vi "Delacor_lib_QMH_Error Handler - Framework Loop.vi"(6 "Error Message Name (\"Error\")":string="Error", 8 "error in":errorcluster, 10 "Ignore Errors (Runtime)":i32[](array[numeric]), 11 "Message Queue in":refnum<class "RQMHMessageQueue.lvclass">) -> (0 "dup error in":errorcluster, 3 "Message Queue out":refnum<class "RQMHMessageQueue.lvclass">)   [LabVIEW 2024, in "RQMHMessageQueue.lvclass"]
doc: "Process an error that occurred in the Event Handling Loop, either by ignoring it, or generating an \"Error\" message.\n____\nDQMH Framework: Palette 7.1.0.1503\nCopyright (c) 2025, DQMH Consortium"
uses:
  RQMHMessageQueue.lvclass
  RQMHMessageQueue.lvclass/RQMHMessageQueue.ctl
  Delacor_lib_QMH_Set Error Debug.vi
  Delacor_lib_QMH_Get Error Debug.vi
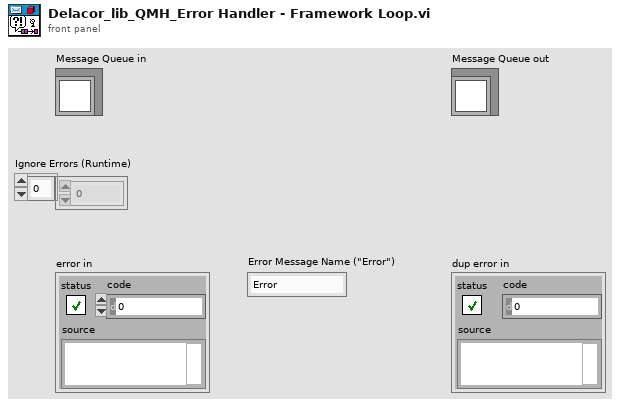
[diagram p1: front panel]
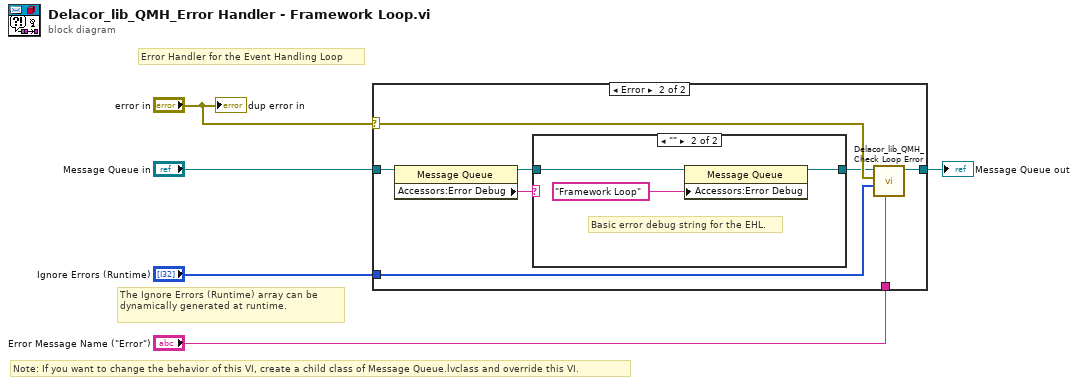
[diagram p0: block diagram]
diagram:
  # "Note: If you want to change the behavior of this VI, create a child class of Message Queue.lvclass and override this VI."
  # "The Ignore Errors (Runtime) array can be dynamically generated at runtime."
  # "Error Handler for the Event Handling Loop"
  n1 = case shown="Error" "error in" {
    selector: "error in" -> [_ w14]
    tunnel: "Message Queue in" -> [w6 w13]
    tunnel: "Ignore Errors (Runtime)" -> [_ w12]
    tunnel: [w6 w11] -> w2
    tunnel: "Error Message Name (\"Error\")" -> [_ w10]
    frame No Error {
    }
    frame Error {
      n2 = property class="Message Queue"(reference=w13) -> (reference out=w8:refnum<class "RQMHMessageQueue.lvclass">, "Accessors:Error Debug"=w7:string)  [unwired: 1 in, 1 out]
      n3 = case shown="\"\"" w7 {
        tunnel: [w15 w18] -> w9
        tunnel: w8 -> [w15 w16]
        frame Default {
          # "(advanced use case) The user has specified a custom Error Debug string via a property node on the message queue class in the EHL. In this case, don't overwrite the string the user has specified."
        }
        frame "" {
          # "Basic error debug string for the EHL."
          n4 = property class="Message Queue"(reference=w16, "Accessors:Error Debug"="Framework Loop") -> (reference out=w18:refnum<class "RQMHMessageQueue.lvclass">)  [unwired: 1 in, 1 out]
        }
      }
      n5 = call-dynamic "Delacor_lib_QMH_Check Loop Error.vi"("Error Message Name (\"Error\")"=w10, "Ignore Errors"=w12, "error to process"=w14, "Message Queue in"=w9) -> ("Message Queue out"=w11:refnum<class "RQMHMessageQueue.lvclass">)  [unwired: 6 in, 1 out]
    }
  }
  "Message Queue out" <- w2
  "dup error in" <- "error in"
